vi "SubtractEYE_MPTool.vi"(0 "Choose Directory":path) -> ()   [LabVIEW 2022 SP3]
uses:
  <vilib>/Analysis/5stat.llb/RMS (DBL).vi
  <vilib>/Analysis/baseanly.llb/Mean (DBL).vi
  <vilib>/Utility/file.llb/Write Delimited Spreadsheet (DBL).vi
  <vilib>/Analysis/NI_AALPro.lvlib
  <vilib>/Analysis/NI_AALBase.lvlib
panel:
  out "Pair 2":sgl[][](graph)
  out "Pair 1":sgl[][](graph)
  out "Array":dbl[][](array[numeric])
  in  "Header format":u16(ring) items=["Riverside Format", "Ron Linear", "GE Bin"]
  in  "Compress":bool
  in  "file ext":string="*.eye"
  out "Current Image":string
  out "Numeric":i32
  in  "Use Selected Files":bool
  in  "Listbox":i32[](listbox)
  # "Slect a batch of eye files and the will be saved as BMP 24 bit RGB. They will be converted to a 1to1 aspect ratio and the batch will be scaled to reflect absolute voltage levels. Data is log compressed. May want to adjust Z scale to improve contrast."
  # "Scale in mm"
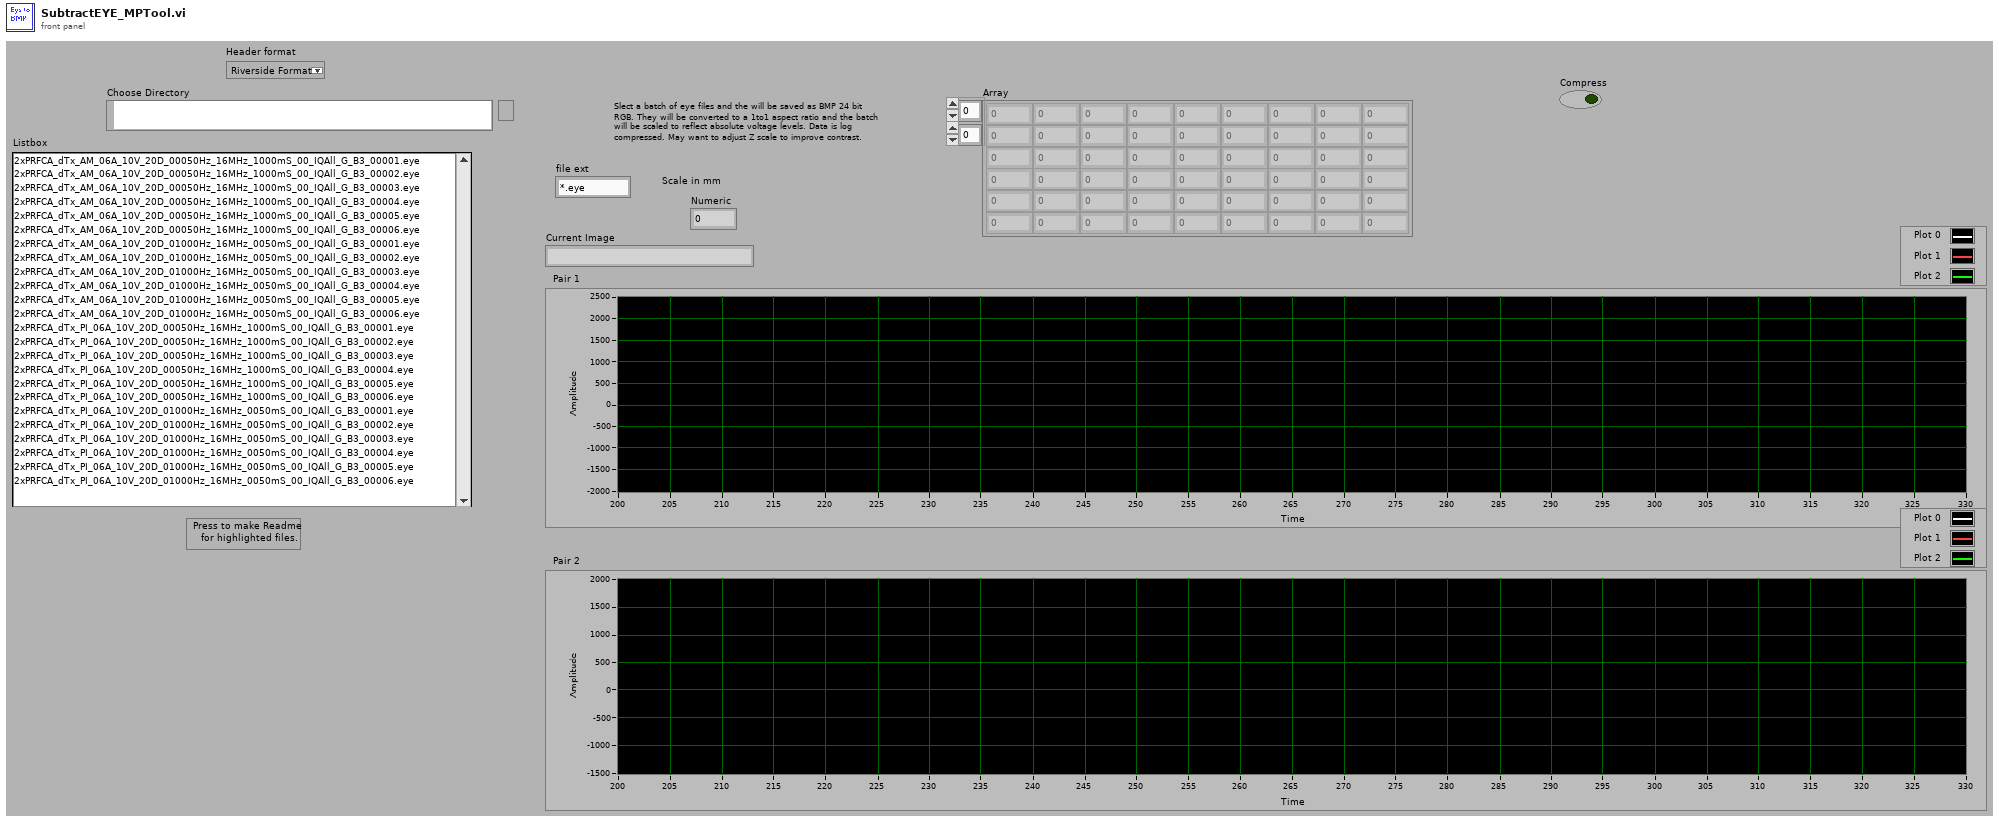
[diagram p1: front panel]
types:
  T1 = typedef "Header.ctl" = cluster{"header info":cluster{"Header":string, "Head length":i16}, "A/D info":cluster{"# rf points per line":u16, "# lines per scan":u16, "sample rate MHz":u16, "# A/D bits":i16, "# bytes per A/D":u16, "TGC Flag":u16, "A/D Type":string}, "Tranducer Info":cluster{"bandwidth":sgl, "center freq":sgl, "start freq":sgl, "ID":i32}, "Scan Info":cluster{"delay":sgl, "pivot distance":sgl, "sector scan angle":sgl, "operator":string, "Scan Mode":string, "location":string}, "Time/Date Info":cluster{"date":string, "time":string}, "RF Info":cluster{"RF file name":string, "RF file att":string, "RF cal file name":string, "RF cal file att":string}, "Patient Info":cluster{"ID":string, "extended ID":string, "age":u16, "sex":string, "previously\nscanned":string, "PSA":sgl, "LOS":u8, "Ethnicty 2":u8, "Race":u8}, "Tissue Type":cluster{"organ":i16, "disease type":i16, "disease location":i16, "IQ_pts":u16, "RcvBuffer":u8, "RcvFrame":u16, "IQBuff":u8, "IQFrame":u16, "IQPage":u8}, "Votage scaling":cluster{"Digitizer (dB)":sgl, "Gain (dB)":sgl, "Atten (dB)":sgl}, "Comment":string, "Misc Info":cluster{"avg num":u16, "c speed":i16, "Div By or SF zones":i16, "XMIT CHS":u8, "RCV CHS":u8, "Xmit angle":sgl}, "Therapy Parameters":cluster{"Theraputic Freq (MHz)":sgl, "Time on (s)":sgl, "Therapy amplitude (mV)":sgl, "Lines Before":u16, "Lines After":u16}, "Scan Settings":cluster{"Energy (uJ or V)":u8, "Damp (Ohm) or Fc":u8, "HP Filt (KHz)":u8, "LP Filt (MHz)":u8, "Gain (db)":u8, "prf (kHz)":sgl, "Distance between\nscan lines (um)":u16, "Distance between\nscan planes (um)":u16, "Scan line gap (um)":sgl, "Scan plane gap (um)":sgl}, "Compression Parameters":cluster{"F1 (MHz)":sgl, "F2 (MHz)":sgl, "% taper":sgl, "duration":sgl}, "Patient Info Xtra":cluster{"First Name":string, "Last Name":string, "Notes":string}, "ROI Box":u16[]}
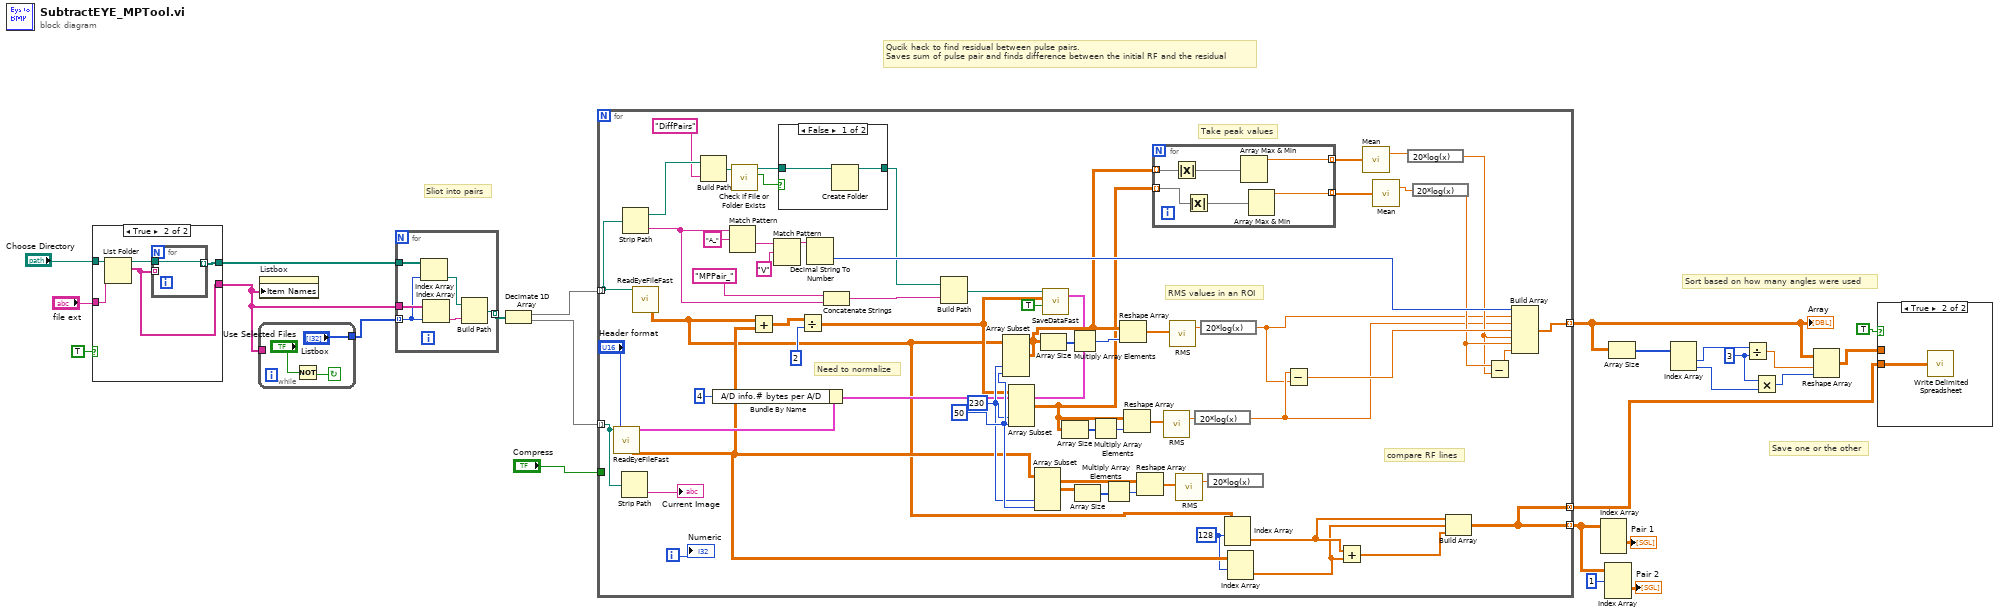
[diagram p0: block diagram]
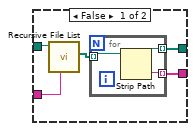
[diagram p4: hidden frame]
diagram:
  w12 = 3 ("y")
  # "Sliot into pairs"
  # "Save one or the other"
  # "Sort based on how many angles were used"
  # "Qucik hack to find residual between pulse pairs.\nSaves sum of pulse pair and finds difference between the initial RF and the residual"
  n1 = case shown="True" TRUE {
    tunnel: [w26 w35] -> w24
    tunnel: "Choose Directory" -> [w29 w37]
    tunnel: [w27 w33] -> w21
    tunnel: "file ext" -> [w25 w36]
    frame False {
      n2 = call <vilib>:"Recursive File List.vi"("pattern"=w25, "Folder Path"=w29) -> ("All Files in Dir"=w28:path[])  [unwired: 5 in, 4 out]
      n3 = for {
        tunnel: w28 -> [w32] mode=indexing
        tunnel: [w31] -> w27 mode=indexing
        tunnel: [w30] -> w26 mode=indexing
        n4 = Strip Path(path=w32) -> (stripped path=w31:path, name=w30:string)
      }
    }
    frame True {
      n5 = List Folder(path=w37, pattern=w36) -> (path out=w34:path, filenames=w35:string[])  [unwired: 1 in, 3 out]
      n6 = for {
        tunnel: w34 -> [w38]
        tunnel: w35 -> [_] mode=indexing
        tunnel: [w38] -> w33 mode=indexing
      }
    }
  }
  n7 = while {
    tunnel: ["Listbox"] -> w23
    tunnel: w24 -> [_]
    stop <- w41 continue-if-true
    n8 = Not(x="Use Selected Files") -> (.not. x?=w41:bool)
  }
  n9 = property on="Listbox" class="LstBox (strict)"("Item Names"=w24) -> ()  [unwired: 2 in, 2 out]
  n10 = for {
    tunnel: w24 -> [w47]
    tunnel: w23 -> [w42] mode=indexing
    tunnel: [w45] -> w17 mode=indexing
    tunnel: w21 -> [w44]
    n11 = Index Array(array=w44, index=w42) -> (element=w43:path)
    n12 = Index Array(array=w47, index=w42) -> (element=w46:string)
    n13 = Build Path(base path=w43, name or relative path=w46) -> (appended path=w45:path)
  }
  n14 = Decimate 1D Array(w17) -> (w15:path[], w16:path[])
  n15 = for {
    tunnel: w16 -> [w109] mode=indexing
    tunnel: "Compress" -> [_]
    tunnel: w15 -> [w105] mode=indexing
    tunnel: [w85] -> w10 mode=indexing
    tunnel: [w48] -> w6 mode=indexing
    tunnel: [w48] -> w2 mode=concatenating
    i -> [w108]
    w53 = 128 ("index (row)")
    w72 = 50 ("length")
    w71 = 230 ("index")
    # "Need to normalize"
    # "Take peak values"
    # "RMS values in an ROI"
    # "compare RF lines"
    n16 = call "ReadEyeFileFast.vi"("new file path"=w109, "Header format"="Header format") -> ("2-D data array"=w54:sgl[][], "Header In"=w57:T1)  [unwired: 16 out]
    n17 = Strip Path(path=w109) -> (name=→"Current Image":string)  [unwired: 1 out]
    n18 = Strip Path(path=w105) -> (stripped path=w63:path, name=w91:string)
    n19 = call "ReadEyeFileFast.vi"("new file path"=w105) -> ("2-D data array"=w51:sgl[][])  [unwired: 1 in, 17 out]
    n20 = Build Path(base path=w63, name or relative path="DiffPairs") -> (appended path=w61:path)
    n21 = Bundle By Name(cluster=w57, "A/D info.# bytes per A/D"=u16 4) -> (w56:T1)
    n22 = Match Pattern(string=w91, regular expression="A_") -> (after substring=w89:string)  [unwired: 1 in, 3 out]
    n23 = call <vilib>:"Check if File or Folder Exists.vi"("path"=w61) -> ("file or folder exists?"=w60:bool, "dup path"=w59:path)  [unwired: 8 in, 1 out]
    n24 = Add(x=w51, y=w54) -> (x+y=w100:sgl[][])
    n25 = Match Pattern(string=w89, regular expression="V") -> (before substring=w87:string)  [unwired: 1 in, 3 out]
    n26 = case shown="False" w60 {
      tunnel: w59 -> [w111 w112]
      tunnel: [w110 w112] -> w58
      frame False {
        n27 = Create Folder(path (use dialog)=w111) -> (created path=w110:path)  [unwired: 2 in, 2 out]
      }
      frame True {
      }
    }
    n28 = Divide(x=w100, y=2) -> (x/y=w65:sgl[][])
    n29 = Decimal String To Number(string=w87) -> (number=w86:i32)  [unwired: 2 in, 1 out]
    n30 = Concatenate Strings("MPPair_" ("string"), w91) -> (w104:string)
    n31 = Build Path(base path=w58, name or relative path=w104) -> (appended path=w102:path)
    n32 = Array Subset(array=w51, index (col)=w71, length (col)=w72) -> (w84:sgl[][])  [unwired: 2 in]
    n33 = Array Subset(array=w65, index (col)=w71, length (col)=w72) -> (w82:sgl[][])  [unwired: 2 in]
    n34 = Array Subset(array=w54, index (col)=w71, length (col)=w72) -> (w66:sgl[][])  [unwired: 2 in]
    n35 = Array Size(array=w84) -> (size(s)=w93:i32[])
    n36 = call "SaveDataFast.vi"("Header In"=w56, "Save?"=TRUE, "Data Array"=w65, "File Name and Path"=w102) -> ()  [unwired: 7 in, 1 out]
    n37 = Array Size(array=w82) -> (size(s)=w97:i32[])
    n38 = Multiply Array Elements(1:w93) -> (0:w96:i32)
    n39 = Array Size(array=w66) -> (size(s)=w68:i32[])
    n40 = Multiply Array Elements(1:w97) -> (0:w99:i32)
    n41 = Multiply Array Elements(1:w68) -> (0:w70:i32)
    n42 = Reshape Array(w84, w96) -> (w94:sgl[])
    n43 = Reshape Array(w82, w99) -> (w83:sgl[])
    n44 = Reshape Array(w66, w70) -> (w67:sgl[])
    n45 = for {
      tunnel: w84 -> [w118] mode=indexing
      tunnel: w82 -> [w117] mode=indexing
      tunnel: [w114] -> w81 mode=indexing
      tunnel: [w113] -> w80 mode=indexing
      n46 = Absolute Value(x=w118) -> (abs(x)=w116:sgl[])
      n47 = Absolute Value(x=w117) -> (abs(x)=w115:sgl[])
      n48 = Array Max & Min(array=w116) -> (max value=w114:sgl)  [unwired: 3 out]
      n49 = Array Max & Min(array=w115) -> (max value=w113:sgl)  [unwired: 3 out]
    }
    n50 = call-poly <vilib>:"RMS.vi"("X"=w83) -> ("rms value"=w98:dbl)  [unwired: 1 out]
    n51 = call-poly <vilib>:"RMS.vi"("X"=w94) -> ("rms value"=w95:dbl)  [unwired: 1 out]
    n52 = call-poly <vilib>:"RMS.vi"("X"=w67) -> ("rms value"=w69:dbl)  [unwired: 1 out]
    n53 = expression code="20*log(x)"(w98) -> (w74:dbl)
    n54 = expression code="20*log(x)"(w95) -> (w73:dbl)
    n55 = expression code="20*log(x)"(w69) -> ()  [unwired: 1 out]
    n56 = Index Array(array=w51, index (row)=w53) -> (element=w50:sgl[])  [unwired: 1 in]
    n57 = Index Array(array=w54, index (row)=w53) -> (element=w49:sgl[])  [unwired: 1 in]
    n58 = Subtract(x=w74, y=w73) -> (x-y=w92:dbl)
    n59 = Add(x=w50, y=w49) -> (x+y=w52:sgl[])
    n60 = call-poly <vilib>:"Mean.vi"("X"=w81) -> ("mean"=w79:dbl)  [unwired: 1 out]
    n61 = call-poly <vilib>:"Mean.vi"("X"=w80) -> ("mean"=w78:dbl)  [unwired: 1 out]
    n62 = expression code="20*log(x)"(w79) -> (w75:dbl)
    n63 = expression code="20*log(x)"(w78) -> (w76:dbl)
    n64 = Build Array(w50, w49, w52) -> (w48:sgl[][])
    n65 = Subtract(x=w76, y=w75) -> (x-y=w77:dbl)
    n66 = Build Array(w86, w73, w74, w92, w75, w76, w77) -> (w85:dbl[])
    "Numeric" <- w108
  }
  "Array" <- w10
  n67 = Index Array(array=w6) -> (element=→"Pair 1":sgl[][])  [unwired: 3 in]
  n68 = Index Array(array=w6, index (dim 0)=1 ("index (page)")) -> (element=→"Pair 2":sgl[][])  [unwired: 2 in]
  n69 = Array Size(array=w10) -> (size(s)=w14:i32[])
  n70 = Index Array(array=w14) -> (element #1=w13:i32, element #2=w11:i32)  [unwired: 2 in]
  n71 = Divide(x=w13, y=w12) -> (x/y=w9:dbl)
  n72 = Multiply(x=w12, y=w11) -> (x*y=w8:i32)
  n73 = Reshape Array(w10, w9, w8) -> (w1:dbl[][])
  n74 = case shown="True" TRUE {
    tunnel: w2 -> [_ w119]
    tunnel: w1 -> [_ _]
    frame False {
    }
    frame True {
      n75 = call-poly <vilib>:"Write Delimited Spreadsheet.vi"("2D data"=w119) -> ()  [unwired: 13 in, 2 out]
    }
  }
